vi "fgt set valve position.vi"(6 "wait (true)":bool=TRUE, 8 "error in (no error)":errorcluster, 9 "direction (shortest)":T1, 10 "position":i32, 11 "valveIndex":u32) -> (0 "error out":errorcluster)   [LabVIEW 2016, in "fgt_SDK.lvlib"]
doc: "Switch valve to the requested position. If Wait is true, block until the valve arrives at the position.\nIf the valve is an M-Switch, the direction input specifies in which direction it should turn."
uses:
  fgt_SDK.lvlib
  TypeDefs/fgt_SWITCH_DIRECTION.ctl
  dlls/fgt_SDK_32.dll
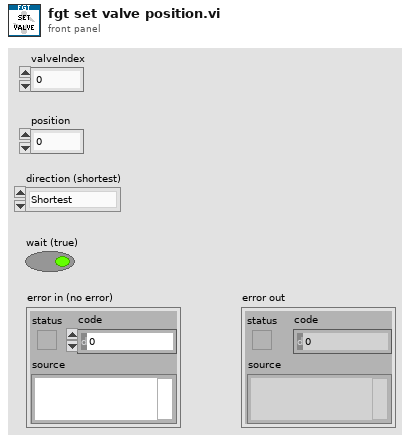
[diagram p1: front panel]
types:
  T1 = typedef "fgt_SDK.lvlib/fgt_SWITCH_DIRECTION.ctl" = enum16{"Shortest", "Anticlockwise", "Clockwise"}
  T2 = typedef "fgt_SDK.lvlib/fgt_STATUS_INFO.ctl" = cluster{"InstrType":T3, "instrSN":u16, "errorCode":u8, "infoCode":u8, "detail":string}
  T3 = typedef "fgt_SDK.lvlib/fgt_INSTRUMENT_TYPE.ctl" = enum32{"None", "MFCS", "MFCS_EZ", "FRP", "LineUP", "IPS"}
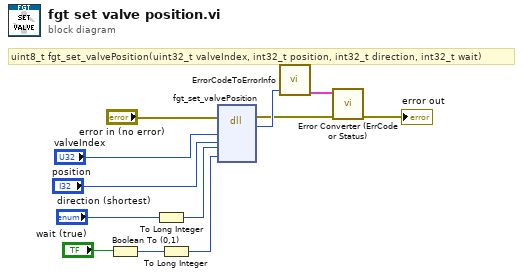
[diagram p0: block diagram]
diagram:
  # "uint8_t fgt_set_valvePosition(uint32_t valveIndex, int32_t position, int32_t direction, int32_t wait)"
  n1 = Boolean To (0,1)(Boolean="wait (true)") -> (0, 1=w8:i16)
  n2 = To Long Integer(number="direction (shortest)") -> (32bit integer=w1:i32)
  n3 = To Long Integer(number=w8) -> (32bit integer=w7:i32)
  n4 = dll-call lib="C:/projects/SDK/fgt-sdk-labview/dlls/fgt_SDK_*.*" fn="fgt_set_valvePosition"(error in="error in (no error)", "valveIndex"="valveIndex", "position"="position", "direction"=w1, "wait"=w7) -> (error out=w4:errorcluster, "return type"=w6:u8)  [unwired: 6 in, 1 out]
  n5 = call "ErrorCodeToErrorInfo.vi"("return type"=w6) -> ("StatusInfo"=w5:T2)  [unwired: 10 in]
  n6 = call "Error Converter (ErrCode or Status).vi"("error in (no error)"=w4, "StatusInfo"=w5) -> ("error out"=→"error out":errorcluster)  [unwired: 9 in]
